vi "Setup Meter Logging.vi"() -> ()   [LabVIEW 2013]
uses:
  <instrlib>/Watts Up Series/Watts Up Series.lvlib
panel:
  in  "Items To Log":bool[](array[boolean])=[TRUE, TRUE, TRUE, TRUE, TRUE, TRUE, TRUE, TRUE, TRUE, TRUE, TRUE, TRUE, TRUE, TRUE, TRUE, TRUE, TRUE, TRUE]
  in  "Threshold (0 W)":dbl
  in  "Rate (0.000 $)":dbl
  in  "Interval (10)":dbl=10.0
  in  "Logging Type (0: Internal)":u16(ring) items=["Internal", "External"]
  in  "VISA resource name":refnum<visa-resource-name>
  # "Watts"
  # "Volts"
  # "Amps"
  # "Watt Hours"
  # "Cost"
  # "WH/Month"
  # "Cost/Month"
  # "Wmax"
  # "Vmax"
  # "Amax"
  # "Wmin"
  # "Vmin"
  # "Amin"
  # "Power Factor"
  # "Duty Cycle"
  # "Power Cycle"
  # "Line Freq."
  # "Volt-Amps"
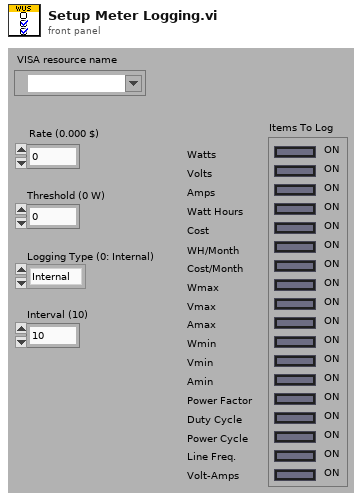
[diagram p1: front panel]
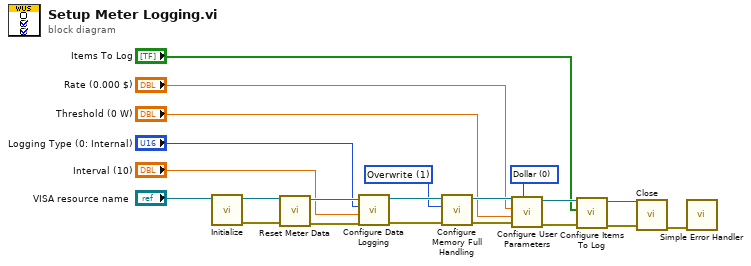
[diagram p0: block diagram]
diagram:
  w14 = u16 0 items=["Dollar", "Euro"] ("Currency (0: Dollar)")
  w18 = u16 1 items=["Stop", "Overwrite", "Automatic"] ("Memory Full Handling Policy (0:Stop)")
  n1 = call <instrlib>:"Initialize.vi"("VISA resource name"="VISA resource name") -> ("error out"=w8:errorcluster, "VISA resource name out"=w9:refnum<visa-resource-name>)  [unwired: 9 in]
  n2 = call <instrlib>:"Reset Meter Data.vi"("error in (no error)"=w8, "VISA resource name"=w9) -> ("error out"=w6:errorcluster, "VISA resource name out"=w7:refnum<visa-resource-name>)  [unwired: 8 in]
  n3 = call <instrlib>:"Configure Data Logging.vi"("error in (no error)"=w6, "Interval (10)"="Interval (10)", "Logging Type (0: Internal)"="Logging Type (0: Internal)", "VISA resource name"=w7) -> ("error out"=w19:errorcluster, "VISA resource name out"=w20:refnum<visa-resource-name>)  [unwired: 6 in]
  n4 = call <instrlib>:"Configure Memory Full Handling.vi"("error in (no error)"=w19, "Memory Full Handling Policy (0:Stop)"=w18, "VISA resource name"=w20) -> ("error out"=w16:errorcluster, "VISA resource name out"=w17:refnum<visa-resource-name>)  [unwired: 7 in]
  n5 = call <instrlib>:"Configure User Parameters.vi"("Currency (0: Dollar)"=w14, "error in (no error)"=w16, "Threshold (0 W)"="Threshold (0 W)", "Rate (0.000 $)"="Rate (0.000 $)", "VISA resource name"=w17) -> ("error out"=w11:errorcluster, "VISA resource name out"=w12:refnum<visa-resource-name>)  [unwired: 5 in]
  n6 = call <instrlib>:"Configure Items To Log.vi"("error in (no error)"=w11, "Items To Log"="Items To Log", "VISA resource name"=w12) -> ("error out"=w2:errorcluster, "VISA resource name out"=w3:refnum<visa-resource-name>)  [unwired: 7 in]
  n7 = call <instrlib>:"Close.vi"("error in (no error)"=w2, "VISA resource name"=w3) -> ("error out"=w1:errorcluster)  [unwired: 9 in]
  n8 = call <vilib>:"Simple Error Handler.vi"("error in (no error)"=w1) -> ()  [unwired: 4 in, 5 out]
